vi "Write Message Stream.vi"(8 "error in (no error)":errorcluster, 10 "Message Stream.lvclass":refnum<class "Message Stream.lvclass">, 11 "Lock-In Remote Actor in":refnum<class "Lock-In Remote Actor.lvclass">) -> (0 "error out":errorcluster, 3 "Lock-In Remote Actor out":refnum<class "Lock-In Remote Actor.lvclass">)   [LabVIEW 2023, in "Lock-In Remote Actor.lvlib" / "Lock-In Remote Actor.lvclass"]
uses:
  Lock-In Remote Actor.lvclass
  <vilib>/ni/Actors/Network Endpoint Actors/Abstract Classes/Message Stream/Message Stream.lvclass
  Lock-In Remote Actor.lvclass/Lock-In Remote Actor.ctl
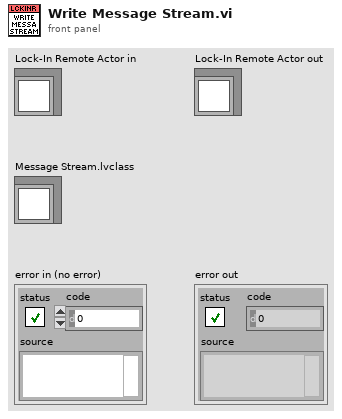
[diagram p1: front panel]
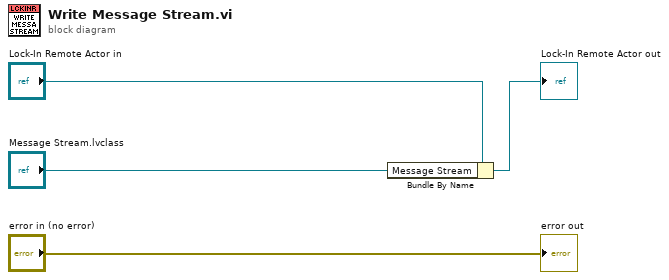
[diagram p0: block diagram]
diagram:
  n1 = Bundle By Name(cluster="Lock-In Remote Actor in", "Message Stream"="Message Stream.lvclass") -> (→"Lock-In Remote Actor out":refnum<class "Lock-In Remote Actor.lvclass">)
  "error out" <- "error in (no error)"
